vi "WS1021 PIC RFFE Cycles.vi"(7 "No of Cycles":i32, 8 "Error In":errorcluster, 10 "Init":bool, 11 "VISA In":refnum<visa-resource-name>) -> (0 "Error Out":errorcluster, 3 "VISA Out":refnum<visa-resource-name>, 5 "Cycles Completed":i32)   [LabVIEW 2017]
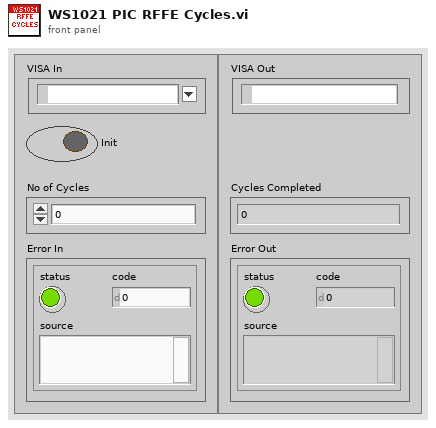
[diagram p1: front panel]
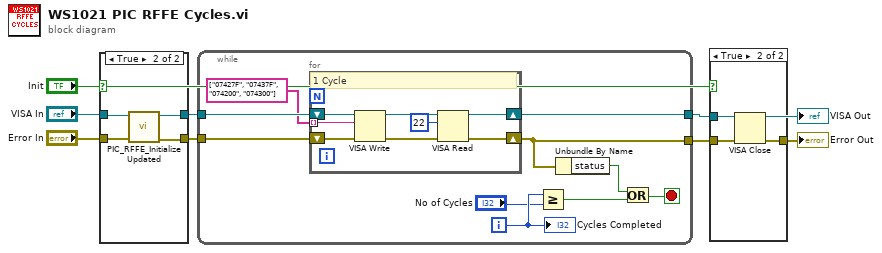
[diagram p0: block diagram]
diagram:
  n1 = case shown="True" "Init" {
    tunnel: "VISA In" -> [w10 w11]
    tunnel: "Error In" -> [w9 w13]
    tunnel: [w9 w14] -> w6
    tunnel: [w10 w12] -> w5
    frame False {
    }
    frame True {
      n2 = call "PIC_RFFE_Initialize Updated.vi"("error in"=w13, "VISA In"=w11) -> ("error out"=w14:errorcluster, "VISA Out"=w12:refnum<visa-resource-name>)  [unwired: 8 in]
    }
  }
  n3 = while {
    tunnel: w6 -> [w23]
    tunnel: w5 -> [w24]
    tunnel: [w19] -> w2
    tunnel: [w18] -> w4
    i -> [w16]
    stop <- w22 stop-if-true
    n4 = for {
      shift-right: [w27] -> w18
      shift-left: w23 -> [w31]
      shift-right: [w28] -> w19
      shift-left: w24 -> [w32]
      tunnel: string[] ["07427F", "07437F", "074200", "074300"] -> [w25] mode=indexing
      # "1 Cycle"
      n5 = VISA Write(VISA resource name=w32, write buffer=w25, error in (no error)=w31) -> (VISA resource name out=w29:refnum<visa-resource-name>, error out=w30:errorcluster)  [unwired: 1 out]
      n6 = VISA Read(VISA resource name=w29, byte count=u32 22, error in (no error)=w30) -> (VISA resource name out=w28:refnum<visa-resource-name>, error out=w27:errorcluster)  [unwired: 2 out]
    }
    n7 = Greater Or Equal?(x=w16, y="No of Cycles") -> (x >= y?=w20:bool)
    n8 = Unbundle By Name(w18) -> ("status"=w21:bool)
    n9 = Or(x=w21, y=w20) -> (x .or. y?=w22:bool)
    "Cycles Completed" <- w16
  }
  "VISA Out" <- w2
  n10 = case shown="True" "Init" {
    tunnel: w4 -> [w33 w36]
    tunnel: [w33 w35] -> w3
    tunnel: w2 -> [_ w34]
    frame False {
    }
    frame True {
      n11 = VISA Close(VISA resource name=w34, error in (no error)=w36) -> (error out=w35:errorcluster)
    }
  }
  "Error Out" <- w3
